vi "XML.GetPropertiesValues.vi"(8 "error in":errorcluster, 9 "rootnode (root of doc)":u32, 10 "property names":string[](array[string]), 11 "XML ref in":u32) -> (0 "error out":errorcluster, 2 "property values":string[](array[string]), 3 "XML ref out":u32)   [LabVIEW 2019, in "Tools.lvlib"]
uses:
  Tools.lvlib
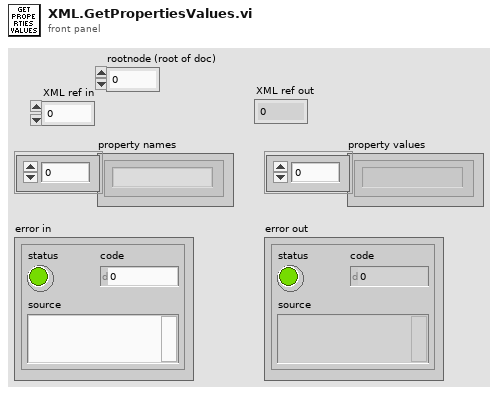
[diagram p1: front panel]
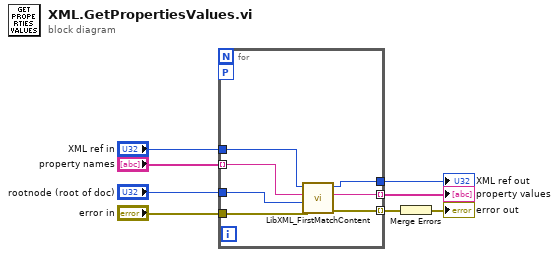
[diagram p0: block diagram]
diagram:
  n1 = for {
    tunnel: "XML ref in" -> [w11]
    tunnel: [w13] -> w7 mode=indexing
    tunnel: [w10] -> w4
    tunnel: "property names" -> [w15] mode=indexing
    tunnel: "error in" -> [w12]
    tunnel: [w14] -> w5 mode=indexing
    workers-P: _ -> [_]
    tunnel: "rootnode (root of doc)" -> [w9]
    n2 = call "LibXML_FirstMatchContent.vi"("error in"=w12, "rootnode (root of doc)"=w9, "xpathexpr"=w15, "doc in"=w11) -> ("error out"=w14:errorcluster, "content"=w13:string, "doc copy out"=w10:u32)  [unwired: 5 in]
  }
  "property values" <- w7
  "XML ref out" <- w4
  n3 = Merge Errors(w5) -> (→"error out":errorcluster)
